vi "Watt.vi"(10 "Current":dbl, 11 "Voltage_in":dbl) -> (3 "Watt":dbl)   [LabVIEW 2013, in "Test_Libraries.lvlib"]
uses:
  Proyecto/Test_Libraries.lvlib
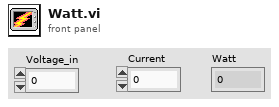
[diagram p1: front panel]
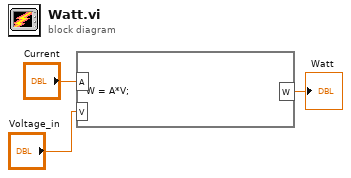
[diagram p0: block diagram]
diagram:
  n1 = formula code="W = A*V;"("A"="Current", "V"="Voltage_in") -> ("W"=→"Watt":dbl)
